vi "Auton_Sl_Shoot_Move.vi"   [LabVIEW 2019]
uses:
  Robot Global Data.vi
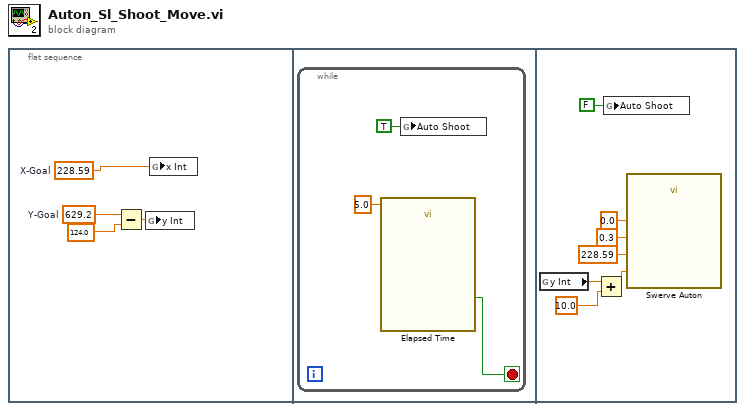
[diagram p0: block diagram]
diagram:
  n1 = flat-sequence {
    frame #0 {
      w4 = 228.59  # X-Goal
      w2 = 629.2  # Y-Goal
      n2 = Subtract(x=w2, y=124.0) -> (x-y=w3:dbl)
      n3 = global write "Robot Global Data.vi" "y Int"(w3) -> ()
      n4 = global write "Robot Global Data.vi" "x Int"(w4) -> ()
    }
    frame #1 {
      n5 = while {
        stop <- w6 stop-if-true
        n6 = call "Elapsed Time"("Time Target (s)"=5.0) -> ("Time has Elapsed"=w6:bool)  [unwired: 11 in, 7 out]
        n7 = global write "Robot Global Data.vi" "Auto Shoot"(TRUE ("Auto Shoot")) -> ()
      }
    }
    frame #2 {
      n8 = global read "Robot Global Data.vi" "y Int"() -> (w10:dbl)
      n9 = Add(x=w10, y=10.0 ("y Distance")) -> (x+y=w9:dbl)
      n10 = global write "Robot Global Data.vi" "Auto Shoot"(FALSE ("Auto Shoot")) -> ()
      n11 = call "Swerve Auton.vi"("Heading"=0.0, "y Distance"=w9, "x Distance"=228.59, "Power"=0.3) -> ()  [unwired: 8 in]
    }
  }
